vi "WSVCAP SHL FPGA LL Procedure RFFE - Clear Lines.vi"(11 "error in (no error)":errorcluster, 13 "Socket Mask":u32) -> (15 "error out":errorcluster)   [LabVIEW 2012]
uses:
  Type Defs/WSVCAP SHL RFFE Write Line Enum.ctl
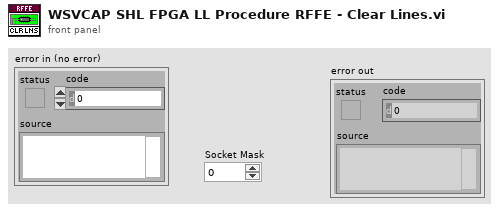
[diagram p1: front panel]
types:
  T1 = typedef "WSVCAP SHL RFFE Write Line Enum.ctl" = enum16{"SDAA", "SCLK"}
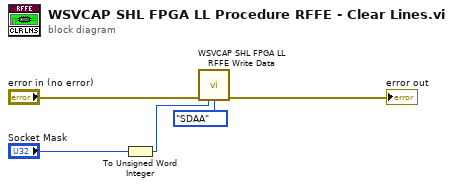
[diagram p0: block diagram]
diagram:
  n1 = To Unsigned Word Integer(number="Socket Mask") -> (unsigned 16bit integer=w4:u16)
  n2 = call "WSVCAP SHL FPGA LL RFFE Write Data.vi"("error in (no error)"="error in (no error)", "Socket Mask"=w4, "Line"=WSVCAP_SHL_RFFE_Write_Line_Enum."SDAA") -> ("error out"=→"error out":errorcluster)  [unwired: 12 in]
